vi "AB_Log_Copy_Source_Item.vi"(4 "loop index":i32, 6 "index":i32, 7 "initial time":u32, 8 "error in (no error)":errorcluster, 9 "newFileFlags":T1, 10 "newFileInfo":T2, 11 "sourcePath":path) -> (0 "error out":errorcluster)   [LabVIEW 2020]
uses:
  <vilib>/AppBuilder/Engine/AB_Engine_New_File_Info.ctl
  <vilib>/AppBuilder/Engine/AB_Engine_New_File_Flags.ctl
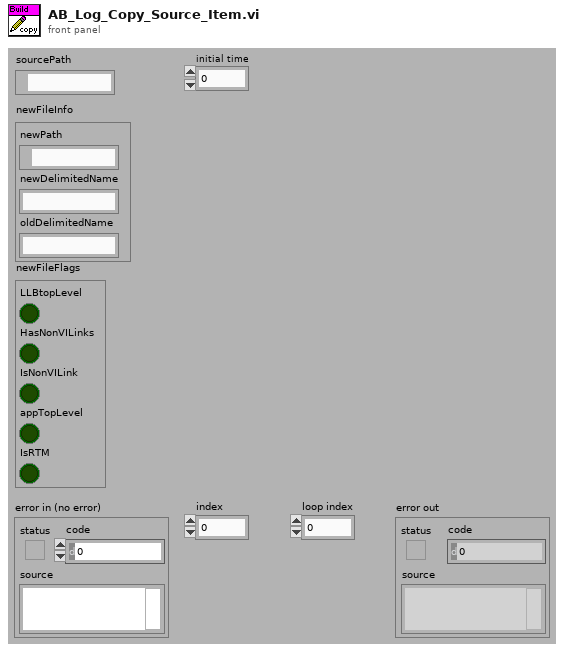
[diagram p1: front panel]
types:
  T1 = typedef "AB_Engine_New_File_Flags.ctl" = cluster{"LLBtopLevel":bool, "HasNonVILinks":bool, "IsNonVILink":bool, "appTopLevel":bool, "IsRTM":bool}
  T2 = typedef "AB_Engine_New_File_Info.ctl" = cluster{"newPath":path, "newDelimitedName":string, "oldDelimitedName":string}
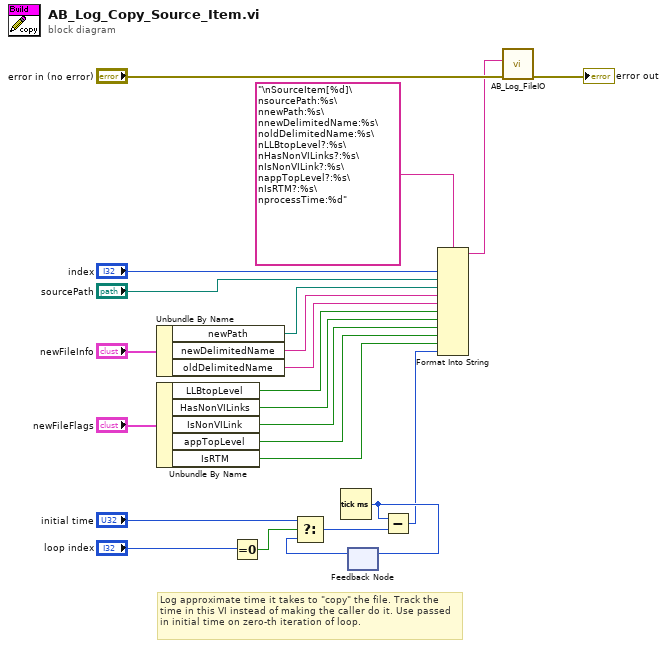
[diagram p0: block diagram]
diagram:
  # "Log approximate time it takes to \"copy\" the file. Track the time in this VI instead of making the caller do it. Use passed in initial time on zero-th iteration of loop."
  n1 = Unbundle By Name("newFileInfo") -> ("newPath"=w10:path, "newDelimitedName"=w9:string, "oldDelimitedName"=w8:string)
  n2 = Unbundle By Name("newFileFlags") -> ("LLBtopLevel"=w7:bool, "HasNonVILinks"=w6:bool, "IsNonVILink"=w5:bool, "appTopLevel"=w4:bool, "IsRTM"=w1:bool)
  n3 = Equal To 0?(x="loop index") -> (x = 0?=w15:bool)
  n4 = Tick Count (ms)() -> (millisecond timer value=w14:u32)
  n5 = feedback-in #1(w14) -> ()
  n6 = feedback #1() -> (w13:u32)  [unwired: 1 out]
  n7 = Select(t="initial time", s=w15, f=w13) -> (s? t:f=w2:u32)
  n8 = Subtract(x=w14, y=w2) -> (x-y=w3:u32)
  n9 = Format Into String(format string="\nSourceItem[%d]\nsourcePath:%s\nnewPath:%s\nnewDelimitedName:%s\noldDelimitedName:%s\nLLBtopLevel?:%s\nHasNonVILinks?:%s\nIsNonVILink?:%s\nappTopLevel?:%s\nIsRTM?:%s\nprocessTime:%d", "index", "sourcePath", w10, w9, w8, w7, w6, w5, w4, w1, w3) -> (resulting string=w11:string)  [unwired: 2 in, 1 out]
  n10 = call <vilib>:"AB_Log_FileIO.vi"("error in (no error)"="error in (no error)", "data"=w11) -> ("error out"=→"error out":errorcluster)  [unwired: 3 in, 6 out]
